vi "Convert Total Flow.vi"(8 "error in (no error)":errorcluster, 9 "3E":u16[](array[numeric]), 10 "3D":u16[](array[numeric]), 11 "3C":u16[](array[numeric]) format="%x") -> (0 "error out":errorcluster, 3 "Totalized Flow (CuFt)":dbl format="%#.4g")   [LabVIEW 2020]
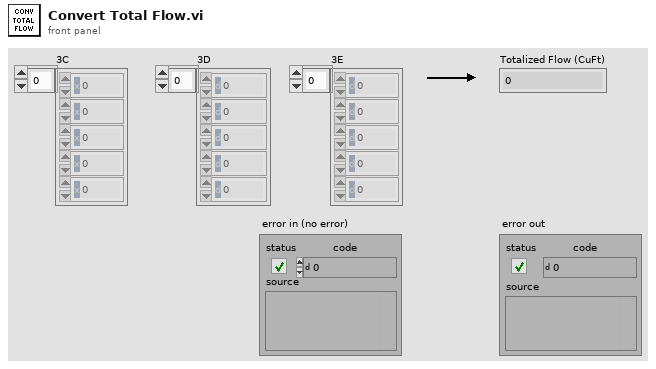
[diagram p1: front panel]
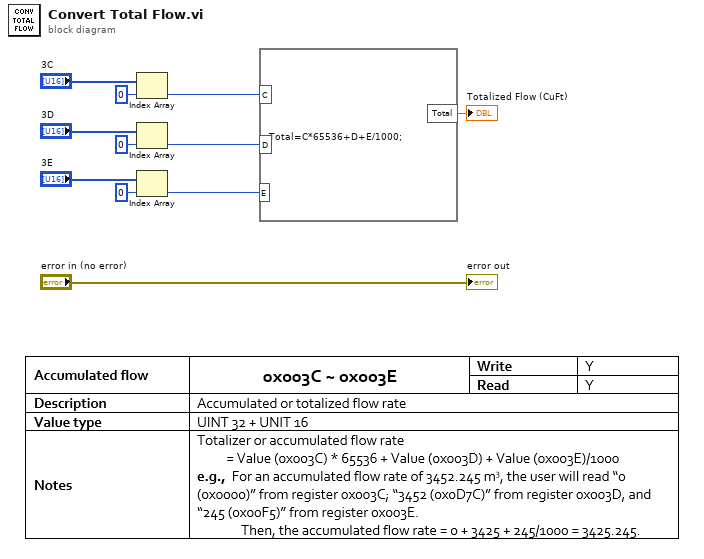
[diagram p0: block diagram]
diagram:
  n1 = Index Array(array="3C", index=0) -> (element=w5:u16)
  n2 = Index Array(array="3D", index=0) -> (element=w4:u16)
  n3 = Index Array(array="3E", index=0) -> (element=w3:u16)
  n4 = formula code="Total=C*65536+D+E/1000;"("C"=w5, "D"=w4, "E"=w3) -> ("Total"=→"Totalized Flow (CuFt)":dbl)
  "error out" <- "error in (no error)"
